vi "Dhoot Front coordinate system.vi"(0 "Image In":T9(plugin-control), 1 "Step Size ROI 1":u32=15, 2 "Scan Direction ROI 1":u16(ring)=2 items=["Left To Right", "Right To Left", "Top To Bottom", "Bottom To Top"], 3 "Search Direction ROI 2":u32, 4 "Line Options ROI 2":T4={"Number of Lines"=1, "Type"=enum."First Edge Rake", "Min. Score"=10.0, "Max. Score"=1000.0, "Orientation"=0.0, "Angle Range"=45.0, "Angle Tolerance"=1.0, "Step Size"=7, "Min. SNR (db)"=0.0, "Min. Points (%)"=25.0, "Hough Iterations"=5} {"Min. Points (%)" min=0.0 max=100.0; "Min. SNR (db)" min=0.0; "Max. Score" min=0.0 max=1024.0; "Min. Score" min=0.0 max=1024.0 step=1.0}, 5 "error in (no error)":errorcluster, 6 "ROI 1":T7 {"Contours"."Type" items=["No Selection", "Point", "Line", "Rectangle", "Oval", "Polygon", "Free", "Annulus", "Unused2", "Unused3", "Broken Line", "Free Hand Line", "Rotated Rectangle"]}, 7 "Edge Options ROI 1":T2={"Edge Polarity"=0, "Kernel Size"=5, "Width"=5, "Minimum Edge Strength"=50.0, "Interpolation Type"=enum."Bilinear Fixed", "Data Processing Method"=enum."Average"} {"Edge Polarity" items=["All Edges", "Rising Edges", "Falling Edges"]; "Minimum Edge Strength" format="%.2f"; "Width" step=2; "Kernel Size" step=2}, 8 "ROI 2":T6 {"Contours"."Type" items=["No Selection", "Point", "Line", "Rectangle", "Oval", "Polygon", "Freehand Region", "Annulus", "Unused2", "Unused3", "Broken Line", "Freehand Line", "Rotated Rectangle"]}, 9 "Edge Options ROI 2":T2={"Edge Polarity"=0, "Kernel Size"=3, "Width"=3, "Minimum Edge Strength"=10.0, "Interpolation Type"=enum."Bilinear Fixed", "Data Processing Method"=enum."Average"} {"Edge Polarity" items=["All Edges", "Rising Edges", "Falling Edges"]; "Minimum Edge Strength" format="%.2f"; "Width" step=2; "Kernel Size" step=2}, 10 "Process ROI 1":T8(ring)=enum."Get First + Last Edge") -> (14 "Co ordinate System":T1, 19 "error out":errorcluster)   [LabVIEW 2019, in "Algorithm.lvclass"]
uses:
  FrameworkOverrides/Algorithm.lvclass
  <vilib>/vision/NI_Vision_Development_Module.lvlib
  <vilib>/vision/Measure.llb/Edge Polarity.ctl
  <vilib>/vision/Measure.llb/Edge Options.ctl
  <vilib>/vision/Measure.llb/Straight Edge Process.ctl
  <vilib>/vision/Measure.llb/Straight Edge Options.ctl
panel:
  out "min value":sgl
  out "Array":sgl[](array[numeric])
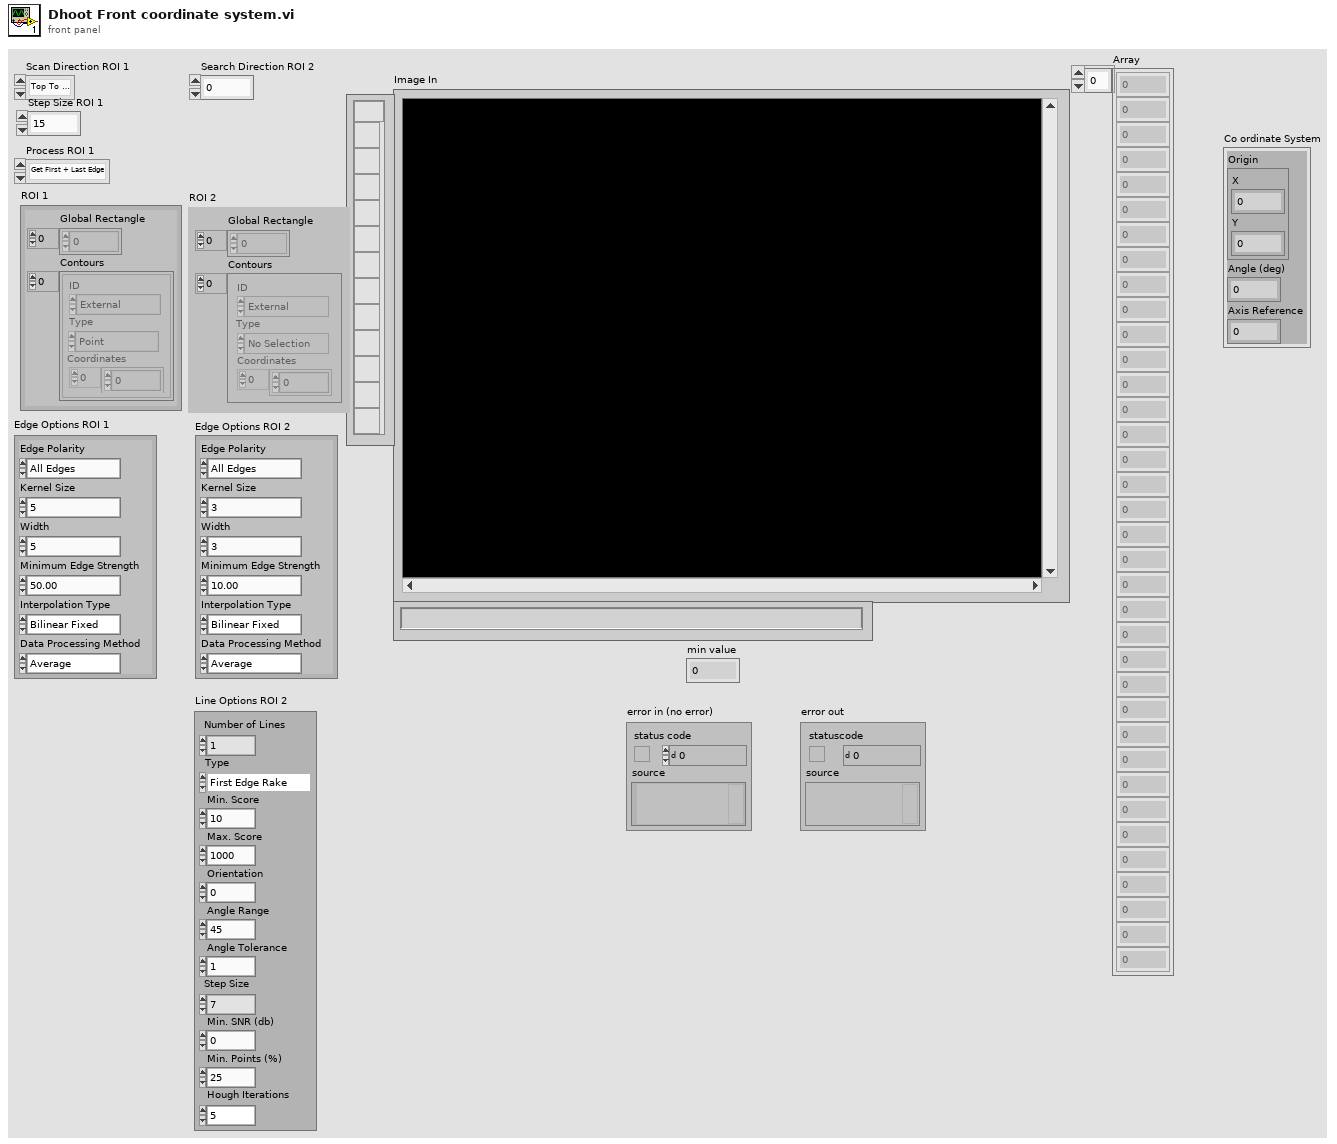
[diagram p1: front panel]
types:
  T1 = cluster{"Origin":cluster{"X":sgl, "Y":sgl}, "Angle (deg)":sgl, "Axis Reference":u32}
  T2 = typedef "Edge Options.ctl" = cluster{"Edge Polarity":T3, "Kernel Size":u32, "Width":u32, "Minimum Edge Strength":sgl, "Interpolation Type":enum32{"Zero Order", "Bilinear", "Quadratic", "Cubic", "Bilinear Fixed"}, "Data Processing Method":enum32{"Average", "Median"}}
  T3 = typedef "Edge Polarity.ctl" = u32
  T4 = typedef "Straight Edge Options.ctl" = cluster{"Number of Lines":i32, "Type":T5, "Min. Score":dbl, "Max. Score":dbl, "Orientation":dbl, "Angle Range":dbl, "Angle Tolerance":dbl, "Step Size":u32, "Min. SNR (db)":dbl, "Min. Points (%)":dbl, "Hough Iterations":i32}
  T5 = typedef "Straight Edge Process.ctl" = enum32{"First Edge Rake", "Best Edge Rake", "Hough Edge Rake", "First Edge Projection", "Best Edge Projection"}
  T6 = typedef "ROI Descriptor" = cluster{"Global Rectangle":i32[], "Contours":cluster{"ID":enum32{"External", "Internal"}, "Type":u32, "Coordinates":i32[]}[]}
  T7 = cluster{"Global Rectangle":i32[], "Contours":cluster{"ID":enum32{"External", "Internal"}, "Type":u32, "Coordinates":i32[]}[]}
  T8 = enum16{"Get First Edge", "Get First + Last Edge", "Get All Edges", "Get Best Edge"}
  T9 = typedef "IMAQ Image.ctl" = refnum<image>
  T10 = cluster{"Search Direction":u32, "Edge Options":T2, "Show Search Area":bool, "Show Search Lines":bool, "Show Edges Found":bool, "Show Result":bool, "Search Area Color":u32, "Search Lines Color":u32, "Edge Locations Color":u32, "Result Color":u32, "Overlay Group Name":string}
  T11 = cluster{"Point 1":cluster{"X":sgl, "Y":sgl}, "Point 2":cluster{"X":sgl, "Y":sgl}}
  T12 = typedef "IMAQ Rectangle" = cluster{"Left":i32, "Top":i32, "Right":i32, "Bottom":i32, "Rotation":dbl}
  T13 = typedef "Edge New.ctl" = cluster{"Location (Pixel)":cluster{"X":sgl, "Y":sgl}, "Location (Real-World)":cluster{"X":sgl, "Y":sgl}, "Distance (Pixel)":dbl, "Distance (Real-World)":dbl, "Strength":dbl, "Noise":dbl, "Rising?":bool}
  T14 = cluster{"Point1 (Pixels)":cluster{"X":sgl, "Y":sgl}, "Point2 (Pixels)":cluster{"X":sgl, "Y":sgl}, "Point1 (Real-World)":cluster{"X":sgl, "Y":sgl}, "Point2 (Real-World)":cluster{"X":sgl, "Y":sgl}, "Angle (Pixel)":dbl, "Angle (Real-World)":dbl, "Score":dbl, "Straightness":dbl, "Average SNR (db)":dbl, "Calibration Valid":bool}[]
  T15 = cluster{"Point1 (Pixels)":cluster{"X":sgl, "Y":sgl}, "Point2 (Pixels)":cluster{"X":sgl, "Y":sgl}, "Point1 (Real-World)":cluster{"X":sgl, "Y":sgl}, "Point2 (Real-World)":cluster{"X":sgl, "Y":sgl}, "Angle (Pixel)":dbl, "Angle (Real-World)":dbl, "Score":dbl, "Straightness":dbl, "Average SNR (db)":dbl, "Calibration Valid":bool}
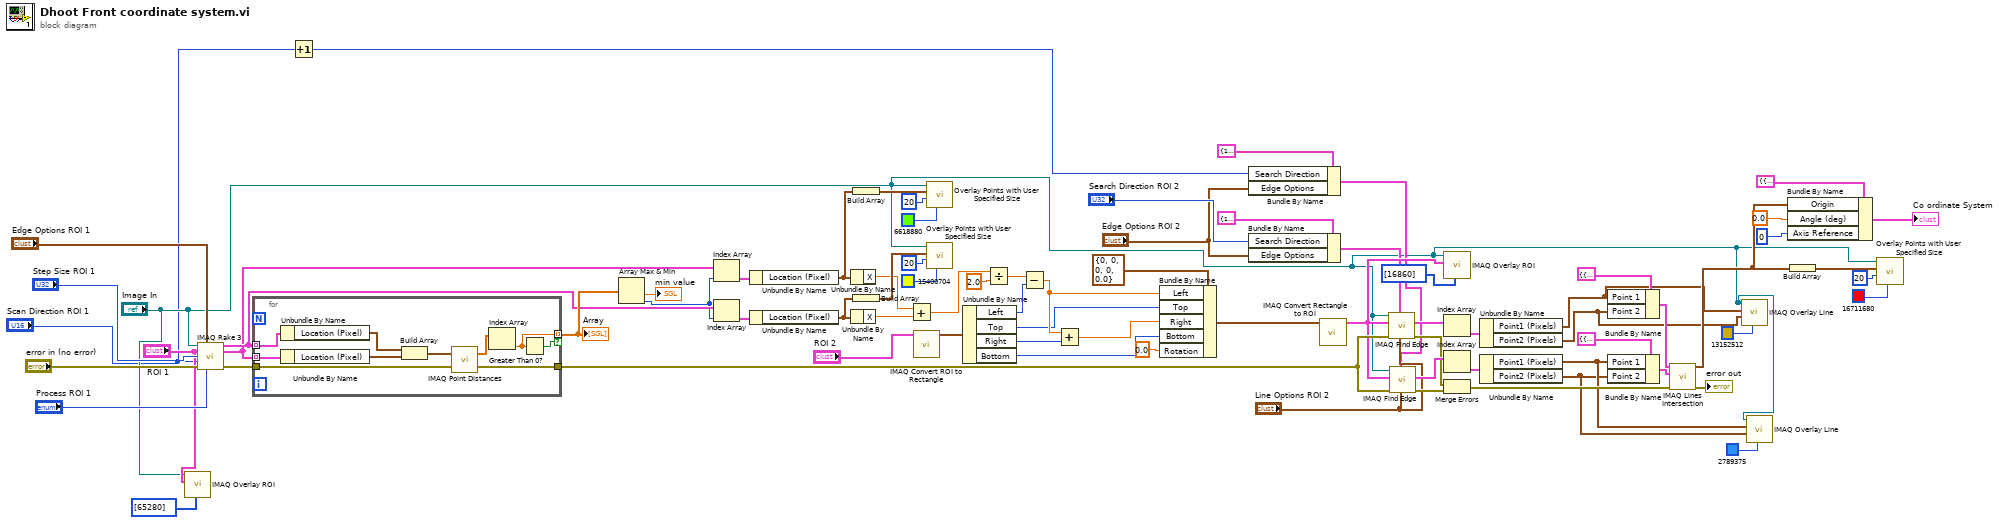
[diagram p0: block diagram]
diagram:
  n1 = call "IMAQ Overlay ROI"("Colors (Green)"=u32[] [65280], "ROI Descriptor"="ROI 1", "Image"="Image In") -> ()  [unwired: 7 in, 2 out]
  n2 = call "IMAQ Rake 3"("Image"="Image In", "Edge Options"="Edge Options ROI 1", "ROI Descriptor"="ROI 1", "Step Size"="Step Size ROI 1", "Scan Direction"="Scan Direction ROI 1", "error in (no error)"="error in (no error)", "Process"="Process ROI 1") -> ("First Edges"=w72:T13[], "Last Edges"=w71:T13[], "error out"=w74:errorcluster)  [unwired: 5 in, 1 out]
  n3 = for {
    tunnel: w72 -> [w87] mode=indexing
    tunnel: w71 -> [w86] mode=indexing
    tunnel: w74 -> [w82]
    tunnel: [w78] -> w73 mode=indexing if=w79
    tunnel: [w80] -> w47
    n4 = Unbundle By Name(w87) -> ("Location (Pixel)"=w85:cluster{"X":sgl, "Y":sgl})
    n5 = Unbundle By Name(w86) -> ("Location (Pixel)"=w84:cluster{"X":sgl, "Y":sgl})
    n6 = Build Array(w85, w84) -> (w83:cluster{"X":sgl, "Y":sgl}[])
    n7 = call "IMAQ Point Distances"("Points"=w83, "error in (no error)"=w82) -> ("Distances"=w81:sgl[], "error out"=w80:errorcluster)  [unwired: 3 in]
    n8 = Index Array(array=w81) -> (element=w78:sgl)  [unwired: 1 in]
    n9 = Greater Than 0?(x=w78) -> (x > 0?=w79:bool)
  }
  "Array" <- w73
  n10 = Increment(x="Scan Direction ROI 1") -> (x+1=w1:u16)
  n11 = Array Max & Min(array=w73) -> (min value=→"min value":sgl, min index (indices)=w62:i32)  [unwired: 2 out]
  n12 = Index Array(array=w71, index=w62) -> (element=w69:T13)
  n13 = Index Array(array=w72, index=w62) -> (element=w70:T13)
  n14 = Unbundle By Name(w69) -> ("Location (Pixel)"=w59:cluster{"X":sgl, "Y":sgl})
  n15 = Unbundle By Name(w70) -> ("Location (Pixel)"=w60:cluster{"X":sgl, "Y":sgl})
  n16 = Unbundle By Name(w59) -> ("X"=w58:sgl)
  n17 = Unbundle By Name(w60) -> ("X"=w57:sgl)
  n18 = Build Array(w59) -> (w67:cluster{"X":sgl, "Y":sgl}[])
  n19 = Build Array(w60) -> (w68:cluster{"X":sgl, "Y":sgl}[])
  n20 = Add(x=w58, y=w57) -> (x+y=w56:sgl)
  n21 = call "IMAQ Convert ROI to Rectangle"("ROI Descriptor"="ROI 2") -> ("Rectangle"=w28:T12)  [unwired: 8 in, 1 out]
  n22 = call "Overlay Points with User Specified Size.vi"("Color"=u32 6618880, "Point Diameter (5)"=u32 20, "Points"=w67, "Image In"="Image In") -> ()  [unwired: 6 in, 2 out]
  n23 = call "Overlay Points with User Specified Size.vi"("Color"=u32 15400704, "Point Diameter (5)"=u32 20, "Points"=w68, "Image In"="Image In") -> ()  [unwired: 6 in, 2 out]
  n24 = Unbundle By Name(w28) -> ("Left"=w27:i32, "Top"=w25:i32, "Right"=w26:i32, "Bottom"=w24:i32)
  n25 = Divide(x=w56, y=sgl 2.0) -> (x/y=w53:sgl)
  n26 = Subtract(x=w53, y=w27) -> (x-y=w52:sgl)
  n27 = Add(x=w52, y=w26) -> (x+y=w51:sgl)
  n28 = Bundle By Name(cluster=T12 {"Left"=0, "Top"=0, "Right"=0, "Bottom"=0, "Rotation"=0.0} ("Rectangle"), "Left"=w52, "Top"=w25, "Right"=w51, "Bottom"=w24, "Rotation"=0.0) -> (w49:T12)
  n29 = Bundle By Name(cluster=T10 {"Search Direction"=1, "Edge Options"={"Edge Polarity"=2, "Kernel Size"=5, "Width"=5, "Minimum Edge Strength"=50.0, "Interpolation Type"=enum."Bilinear Fixed", "Data Processing Method"=enum."Average"}, "Show Search Area"=FALSE, "Show Search Lines"=FALSE, "Show Edges Found"=FALSE, "Show Result"=TRUE, "Search Area Color"=65280, "Search Lines Color"=255, "Edge Locations Color"=16776960, "Result Color"=16711680, "Overlay Group Name"=""} ("Options"), "Search Direction"=w1, "Edge Options"="Edge Options ROI 2") -> (w10:T10)
  n30 = Bundle By Name(cluster=T10 {"Search Direction"=1, "Edge Options"={"Edge Polarity"=2, "Kernel Size"=5, "Width"=5, "Minimum Edge Strength"=50.0, "Interpolation Type"=enum."Bilinear Fixed", "Data Processing Method"=enum."Average"}, "Show Search Area"=FALSE, "Show Search Lines"=FALSE, "Show Edges Found"=FALSE, "Show Result"=TRUE, "Search Area Color"=65280, "Search Lines Color"=255, "Edge Locations Color"=16776960, "Result Color"=16711680, "Overlay Group Name"=""} ("Options"), "Search Direction"="Search Direction ROI 2", "Edge Options"="Edge Options ROI 2") -> (w22:T10)
  n31 = call "IMAQ Convert Rectangle to ROI"("Rectangle"=w49) -> ("ROI Descriptor"=w46:T6)  [unwired: 8 in, 1 out]
  n32 = call "IMAQ Find Edge"("Line Fit Options"="Line Options ROI 2", "Options"=w22, "error in (no error)"=w47, "ROI Descriptor"=w46, "Image"="Image In") -> ("error out"=w36:errorcluster, "Straight Edges"=w45:T14)  [unwired: 3 in, 2 out]
  n33 = call "IMAQ Find Edge"("Line Fit Options"="Line Options ROI 2", "Options"=w10, "error in (no error)"=w47, "ROI Descriptor"=w46, "Image"="Image In") -> ("error out"=w35:errorcluster, "Straight Edges"=w44:T14)  [unwired: 3 in, 2 out]
  n34 = call "IMAQ Overlay ROI"("Colors (Green)"=u32[] [16860], "ROI Descriptor"=w46, "Image"="Image In") -> ()  [unwired: 7 in, 2 out]
  n35 = Index Array(array=w45) -> (element=w43:T15)  [unwired: 1 in]
  n36 = Index Array(array=w44) -> (element=w42:T15)  [unwired: 1 in]
  n37 = Merge Errors(w36, w35) -> (w34:errorcluster)
  n38 = Unbundle By Name(w43) -> ("Point1 (Pixels)"=w9:cluster{"X":sgl, "Y":sgl}, "Point2 (Pixels)"=w8:cluster{"X":sgl, "Y":sgl})
  n39 = Unbundle By Name(w42) -> ("Point1 (Pixels)"=w5:cluster{"X":sgl, "Y":sgl}, "Point2 (Pixels)"=w4:cluster{"X":sgl, "Y":sgl})
  n40 = Bundle By Name(cluster=T11 {"Point 1"={"X"=0.0, "Y"=0.0}, "Point 2"={"X"=0.0, "Y"=0.0}} ("Line 1"), "Point 1"=w9, "Point 2"=w8) -> (w39:T11)
  n41 = Bundle By Name(cluster=T11 {"Point 1"={"X"=0.0, "Y"=0.0}, "Point 2"={"X"=0.0, "Y"=0.0}} ("Line 1"), "Point 1"=w5, "Point 2"=w4) -> (w38:T11)
  n42 = call "IMAQ Lines Intersection"("error in (no error)"=w34, "Line 2"=w38, "Line 1"=w39) -> ("error out"=→"error out":errorcluster, "Intersection Point"=w16:cluster{"X":sgl, "Y":sgl})  [unwired: 6 in, 1 out]
  n43 = call "IMAQ Overlay Line"("Color"=u32 13152512, "End Point"=w8, "Start Point"=w9, "Image"="Image In") -> ()  [unwired: 6 in, 2 out]
  n44 = call "IMAQ Overlay Line"("Color"=u32 2789375, "End Point"=w4, "Start Point"=w5, "Image"="Image In") -> ()  [unwired: 6 in, 2 out]
  n45 = Bundle By Name(cluster=T1 {"Origin"={"X"=0.0, "Y"=0.0}, "Angle (deg)"=0.0, "Axis Reference"=0} ("Coordinate System"), "Origin"=w16, "Angle (deg)"=sgl 0.0, "Axis Reference"=u32 0) -> (→"Co ordinate System":T1)
  n46 = Build Array(w16) -> (w37:cluster{"X":sgl, "Y":sgl}[])
  n47 = call "Overlay Points with User Specified Size.vi"("Color"=u32 16711680, "Point Diameter (5)"=u32 20, "Points"=w37, "Image In"="Image In") -> ()  [unwired: 6 in, 2 out]
